vi "SumoBot.vi"   [LabVIEW 2016, in "SumoRobot.lvrbt"]
uses:
  SumoRobot.lvrbt
  <vilib>/NXT/Block Support/NXT_InputPort.ctl
  <vilib>/NXT/Block Support/NXT_OutputPort.ctl
  <vilib>/NXT/Dual Mode Library/Sensors/EV3_Color_Reflect.vi
  <vilib>/NXT/NXTIO Xnodes/NXTIONodeSubVIs/NXTMoveMotors.vi
  <vilib>/NXT/Dual Mode Library/Sensors/EV3_Ultrasonic_IN.vi
  <vilib>/NXT/Subs/LVHSConnector.ctl
  <vilib>/NXT/NXTIO Xnodes/AddressXNode/NXTIOAddress.xnode
  <vilib>/NXT/NXTIO Xnodes/NXTIOXNode/NXTIO.xnode
  <vilib>/NXT/LegoClasses/BrickReference/BrickReference.lvclass
types:
  T1 = typedef "NXT_InputPort.ctl" = u32
  T2 = typedef "NXT_OutputPort.ctl" = u8
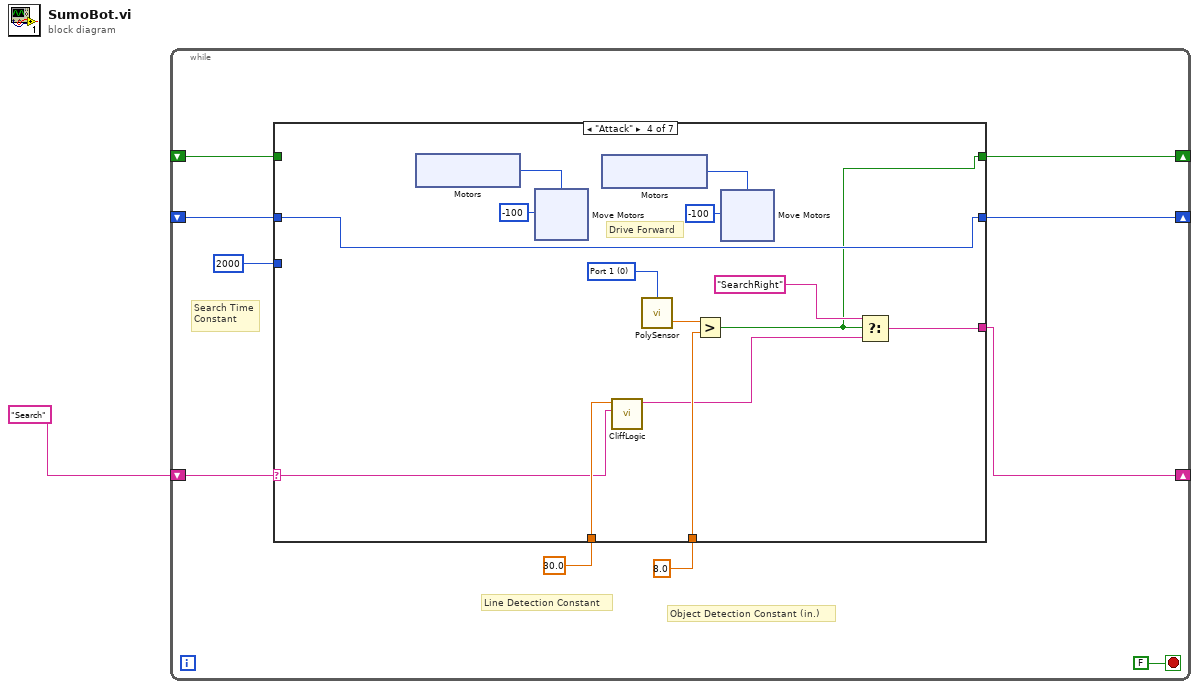
[diagram p0: block diagram]
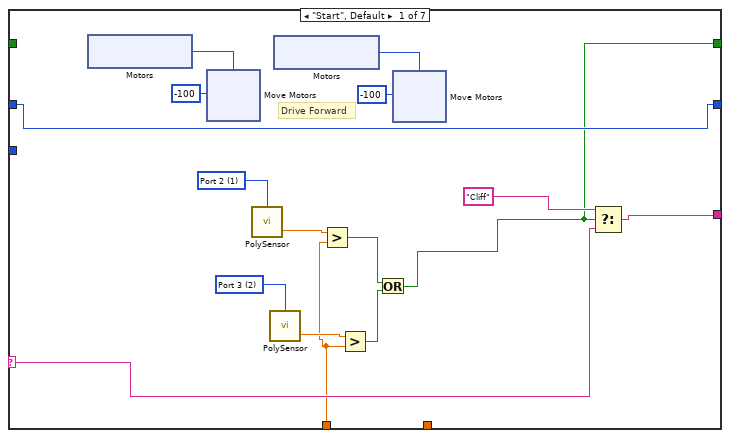
[diagram p2: hidden frame]
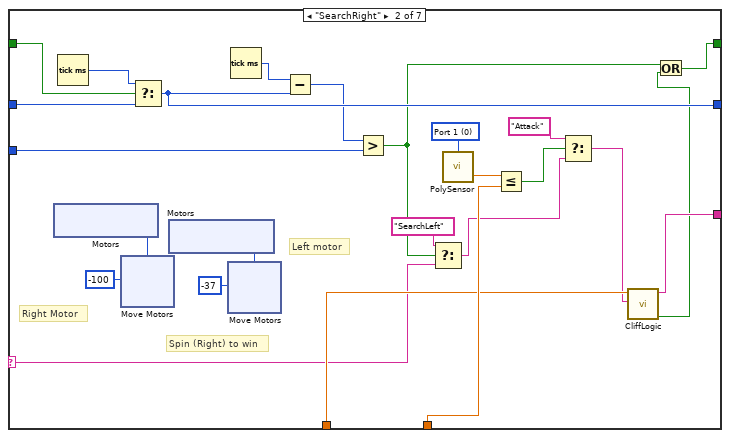
[diagram p3: hidden frame]
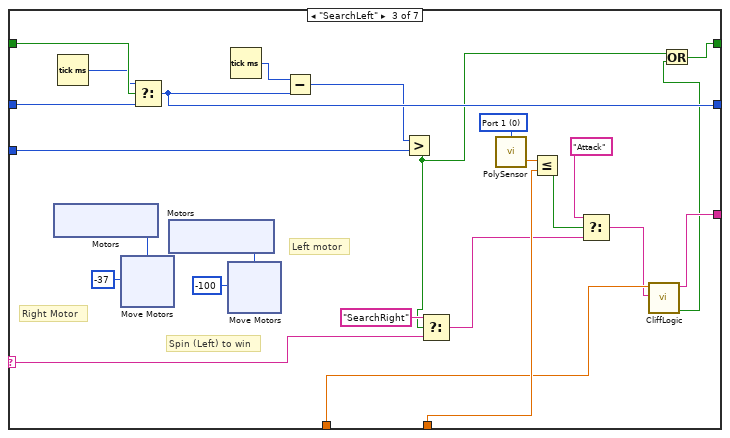
[diagram p4: hidden frame]
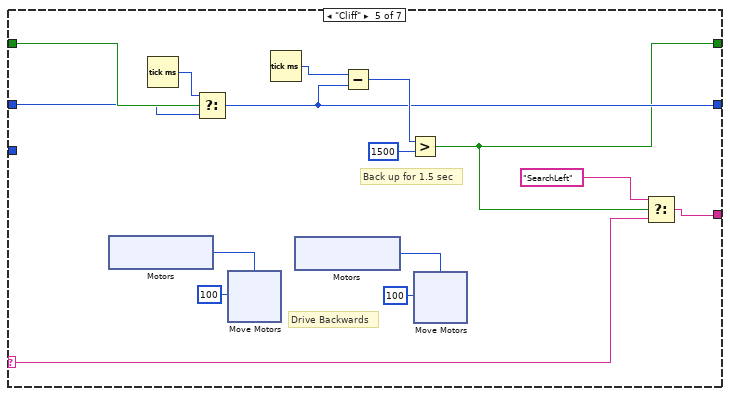
[diagram p5: hidden frame]
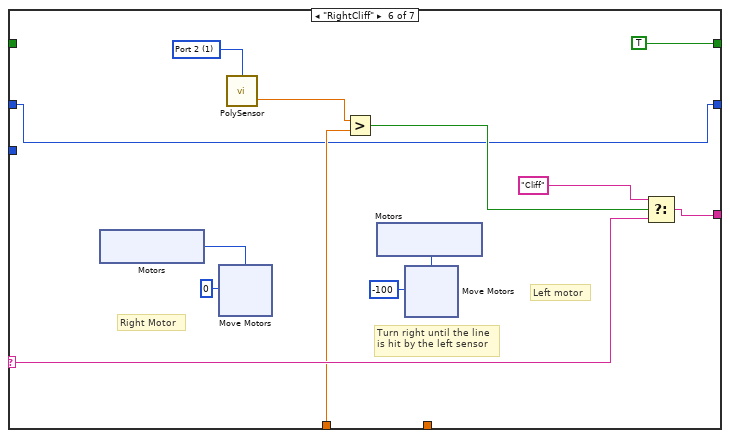
[diagram p6: hidden frame]
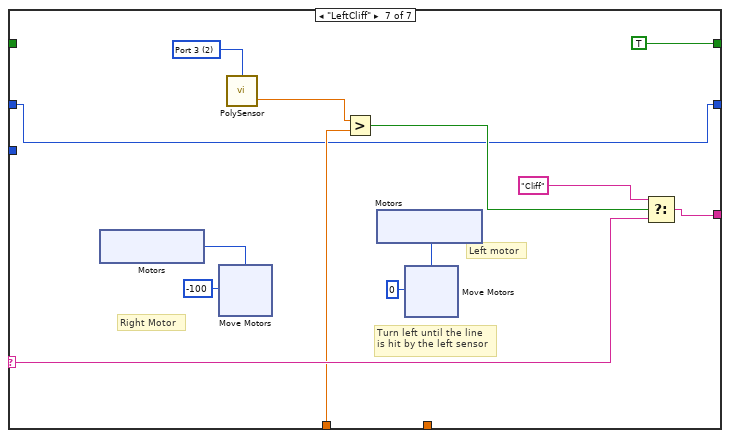
[diagram p7: hidden frame]
diagram:
  n1 = while {
    shift-right: [w7] -> _
    shift-left: "Search" -> [w10]
    shift-right: [w6] -> _
    shift-left: _ -> [w5]
    shift-right: [w4] -> _
    shift-left: _ -> [w3]
    stop <- FALSE stop-if-true
    # "Search Time\nConstant"
    # "Object Detection Constant (in.)"
    # "Line Detection Constant"
    n2 = case shown="\"Attack\"" w10 {
      selector: w10 -> [w22 w50 w91 w127 w167 w198 w227]
      tunnel: sgl 8.0 ("y") -> [_ w62 w103 w130 _ _ _]
      tunnel: sgl 30.0 ("y") -> [w13 w59 w100 w128 _ w190 w219]
      tunnel: [w21 w47 w88 w132 w166 w197 w226] -> w7
      tunnel: [w12 w44 w86 w126 w156 TRUE TRUE] -> w6
      tunnel: w5 -> [_ w57 w98 _ w159 _ _]
      tunnel: [w20 w54 w95 w131 w157 w187 w216] -> w4
      tunnel: w3 -> [w20 w55 w96 w131 w158 w187 w216]
      tunnel: u32 2000 ("y") -> [_ w52 w93 _ _ _ _]
      frame "Start", Default {
        w16 = T1 2 items=["Port 1", "Port 2", "Port 3", "Port 4"] ("Port (Port 1)")
        w19 = T1 1 items=["Port 1", "Port 2", "Port 3", "Port 4"] ("Port (Port 1)")
        # "Drive Forward"
        n3 = xnode "Motors"() -> ("Motor"=w27:T2)
        n4 = xnode "Move Motors"("Power/Speed 1"=i8 -100, "Motors"=w27) -> ()  [unwired: 1 in, 1 out]
        n5 = call-poly <vilib>:"PolySensor.vi"("Port (Port 1)"=w19) -> ("Scaled Value"=w18:sgl)  [unwired: 2 in, 1 out]
        n6 = call-poly <vilib>:"PolySensor.vi"("Port (Port 1)"=w16) -> ("Scaled Value"=w17:sgl)  [unwired: 2 in, 1 out]
        n7 = xnode "Motors"() -> ("Motor"=w24:T2)
        n8 = Greater?(x=w18, y=w13) -> (0:w15:bool)
        n9 = Greater?(x=w17, y=w13) -> (0:w14:bool)
        n10 = Or(x=w15, y=w14) -> (x .or. y?=w12:bool)
        n11 = xnode "Move Motors"("Power/Speed 1"=i8 -100, "Motors"=w24) -> ()  [unwired: 1 in, 1 out]
        n12 = Select(t="Cliff", s=w12, f=w22) -> (s? t:f=w21:string)
      }
      frame "SearchRight" {
        w64 = T1 0 items=["Port 1", "Port 2", "Port 3", "Port 4"] ("Port (Port 1)")
        # "Right Motor"
        # "Left motor"
        # "Spin (Right) to win"
        n13 = xnode "Motors"() -> ("Motor"=w68:T2)
        n14 = Tick Count (ms)() -> (millisecond timer value=w56:u32)
        n15 = xnode "Move Motors"("Power/Speed 1"=i8 -100, "Motors"=w68) -> ()  [unwired: 1 in, 1 out]
        n16 = Select(t=w56, s=w57, f=w55) -> (s? t:f=w54:u32)
        n17 = xnode "Motors"() -> ("Motor"=w65:T2)
        n18 = xnode "Move Motors"("Power/Speed 1"=i8 -37, "Motors"=w65) -> ()  [unwired: 1 in, 1 out]
        n19 = Tick Count (ms)() -> (millisecond timer value=w58:u32)
        n20 = Subtract(x=w58, y=w54) -> (x-y=w53:u32)
        n21 = Greater?(x=w53, y=w52) -> (0:w45:bool)
        n22 = Select(t="SearchLeft", s=w45, f=w50) -> (s? t:f=w49:string)
        n23 = call-poly <vilib>:"PolySensor.vi"("Port (Port 1)"=w64) -> ("Inches"=w63:sgl)  [unwired: 2 in, 1 out]
        n24 = Less Or Equal?(x=w63, y=w62) -> (x <= y?=w61:bool)
        n25 = Select(t="Attack", s=w61, f=w49) -> (s? t:f=w48:string)
        n26 = call "CliffLogic.vi"("State In"=w48, "Light Threshold"=w59) -> ("Both Light"=w46:bool, "State Out"=w47:string)  [unwired: 6 in, 2 out]
        n27 = Or(x=w45, y=w46) -> (x .or. y?=w44:bool)
      }
      frame "SearchLeft" {
        w105 = T1 0 items=["Port 1", "Port 2", "Port 3", "Port 4"] ("Port (Port 1)")
        # "Right Motor"
        # "Left motor"
        # "Spin (Left) to win"
        n28 = xnode "Motors"() -> ("Motor"=w109:T2)
        n29 = Tick Count (ms)() -> (millisecond timer value=w97:u32)
        n30 = xnode "Move Motors"("Power/Speed 1"=i8 -37, "Motors"=w109) -> ()  [unwired: 1 in, 1 out]
        n31 = Select(t=w97, s=w98, f=w96) -> (s? t:f=w95:u32)
        n32 = xnode "Motors"() -> ("Motor"=w106:T2)
        n33 = xnode "Move Motors"("Power/Speed 1"=i8 -100, "Motors"=w106) -> ()  [unwired: 1 in, 1 out]
        n34 = Tick Count (ms)() -> (millisecond timer value=w99:u32)
        n35 = Subtract(x=w99, y=w95) -> (x-y=w94:u32)
        n36 = Greater?(x=w94, y=w93) -> (0:w85:bool)
        n37 = Select(t="SearchRight", s=w85, f=w91) -> (s? t:f=w90:string)
        n38 = call-poly <vilib>:"PolySensor.vi"("Port (Port 1)"=w105) -> ("Inches"=w104:sgl)  [unwired: 2 in, 1 out]
        n39 = Less Or Equal?(x=w104, y=w103) -> (x <= y?=w102:bool)
        n40 = Select(t="Attack", s=w102, f=w90) -> (s? t:f=w89:string)
        n41 = call "CliffLogic.vi"("State In"=w89, "Light Threshold"=w100) -> ("Both Light"=w87:bool, "State Out"=w88:string)  [unwired: 6 in, 2 out]
        n42 = Or(x=w85, y=w87) -> (x .or. y?=w86:bool)
      }
      frame "Attack" {
        w135 = T1 0 items=["Port 1", "Port 2", "Port 3", "Port 4"] ("Port (Port 1)")
        # "Drive Forward"
        n43 = xnode "Motors"() -> ("Motor"=w139:T2)
        n44 = xnode "Move Motors"("Power/Speed 1"=i8 -100, "Motors"=w139) -> ()  [unwired: 1 in, 1 out]
        n45 = xnode "Motors"() -> ("Motor"=w136:T2)
        n46 = call "CliffLogic.vi"("State In"=w127, "Light Threshold"=w128) -> ("State Out"=w129:string)  [unwired: 6 in, 3 out]
        n47 = call-poly <vilib>:"PolySensor.vi"("Port (Port 1)"=w135) -> ("Inches"=w134:sgl)  [unwired: 2 in, 1 out]
        n48 = Greater?(x=w134, y=w130) -> (0:w126:bool)
        n49 = xnode "Move Motors"("Power/Speed 1"=i8 -100, "Motors"=w136) -> ()  [unwired: 1 in, 1 out]
        n50 = Select(t="SearchRight", s=w126, f=w129) -> (s? t:f=w132:string)
      }
      frame "Cliff" {
        # "Drive Backwards"
        # "Back up for 1.5 sec"
        n51 = xnode "Motors"() -> ("Motor"=w164:T2)
        n52 = Tick Count (ms)() -> (millisecond timer value=w160:u32)
        n53 = Select(t=w160, s=w159, f=w158) -> (s? t:f=w157:u32)
        n54 = xnode "Move Motors"("Power/Speed 1"=i8 100, "Motors"=w164) -> ()  [unwired: 1 in, 1 out]
        n55 = Tick Count (ms)() -> (millisecond timer value=w170:u32)
        n56 = xnode "Motors"() -> ("Motor"=w161:T2)
        n57 = Subtract(x=w170, y=w157) -> (x-y=w169:u32)
        n58 = Greater?(x=w169, y=u32 1500) -> (0:w156:bool)
        n59 = xnode "Move Motors"("Power/Speed 1"=i8 100, "Motors"=w161) -> ()  [unwired: 1 in, 1 out]
        n60 = Select(t="SearchLeft", s=w156, f=w167) -> (s? t:f=w166:string)
      }
      frame "RightCliff" {
        w191 = T1 1 items=["Port 1", "Port 2", "Port 3", "Port 4"] ("Port (Port 1)")
        # "Right Motor"
        # "Left motor"
        # "Turn right until the line\nis hit by the left sensor"
        n61 = xnode "Motors"() -> ("Motor"=w195:T2)
        n62 = xnode "Move Motors"("Power/Speed 1"=i8 0, "Motors"=w195) -> ()  [unwired: 1 in, 1 out]
        n63 = call-poly <vilib>:"PolySensor.vi"("Port (Port 1)"=w191) -> ("Scaled Value"=w189:sgl)  [unwired: 2 in, 1 out]
        n64 = Greater?(x=w189, y=w190) -> (0:w188:bool)
        n65 = xnode "Motors"() -> ("Motor"=w192:T2)
        n66 = xnode "Move Motors"("Power/Speed 1"=i8 -100, "Motors"=w192) -> ()  [unwired: 1 in, 1 out]
        n67 = Select(t="Cliff", s=w188, f=w198) -> (s? t:f=w197:string)
      }
      frame "LeftCliff" {
        w220 = T1 2 items=["Port 1", "Port 2", "Port 3", "Port 4"] ("Port (Port 1)")
        # "Right Motor"
        # "Left motor"
        # "Turn left until the line\nis hit by the left sensor"
        n68 = xnode "Motors"() -> ("Motor"=w224:T2)
        n69 = xnode "Move Motors"("Power/Speed 1"=i8 -100, "Motors"=w224) -> ()  [unwired: 1 in, 1 out]
        n70 = call-poly <vilib>:"PolySensor.vi"("Port (Port 1)"=w220) -> ("Scaled Value"=w218:sgl)  [unwired: 2 in, 1 out]
        n71 = Greater?(x=w218, y=w219) -> (0:w217:bool)
        n72 = xnode "Motors"() -> ("Motor"=w221:T2)
        n73 = xnode "Move Motors"("Power/Speed 1"=i8 0, "Motors"=w221) -> ()  [unwired: 1 in, 1 out]
        n74 = Select(t="Cliff", s=w217, f=w227) -> (s? t:f=w226:string)
      }
    }
  }
